vi "Prins FIFO Scheduler.vi"(8 "Number of Jobs":i32=4, 9 "Number of Machines":i32=4, 10 "Processing Times(MxJ)":u16[][](array[numeric])=[[1, 62, 270, 667], [303, 255, 170, 272], [66, 556, 373, 5], [630, 127, 187, 56]], 11 "Schedule In":u16[](array[numeric])=[6, 12, 5, 1, 10, 15, 4, 0, 14, 7, 13, 3, 2, 8, 11, 9]) -> (2 "Completion Times (MxJ)":i32[][](array[numeric]), 3 "Start Times (MxJ)":i32[][](array[numeric]))   [LabVIEW 2013, in "Scheduler.lvclass"]
uses:
  Scheduler.lvclass
  Controls/GapStructure4FIFOEngine.ctl
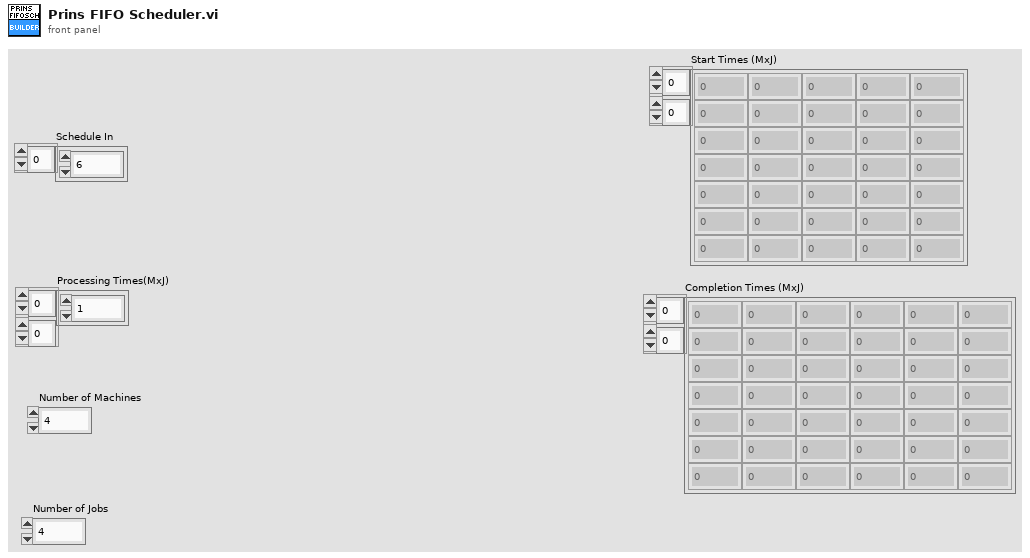
[diagram p1: front panel]
types:
  T1 = typedef "Scheduler.lvclass/GapStructure4FIFOEngine.ctl" = cluster{"Gap Start":i32, "Gap End":i32, "Gap Valid?":bool}
  T2 = typedef "Scheduler.lvclass/ValidGaps.ctl" = cluster{"Gap Start Time":i32, "Gap End Time":i32, "Gap Interval":i32}
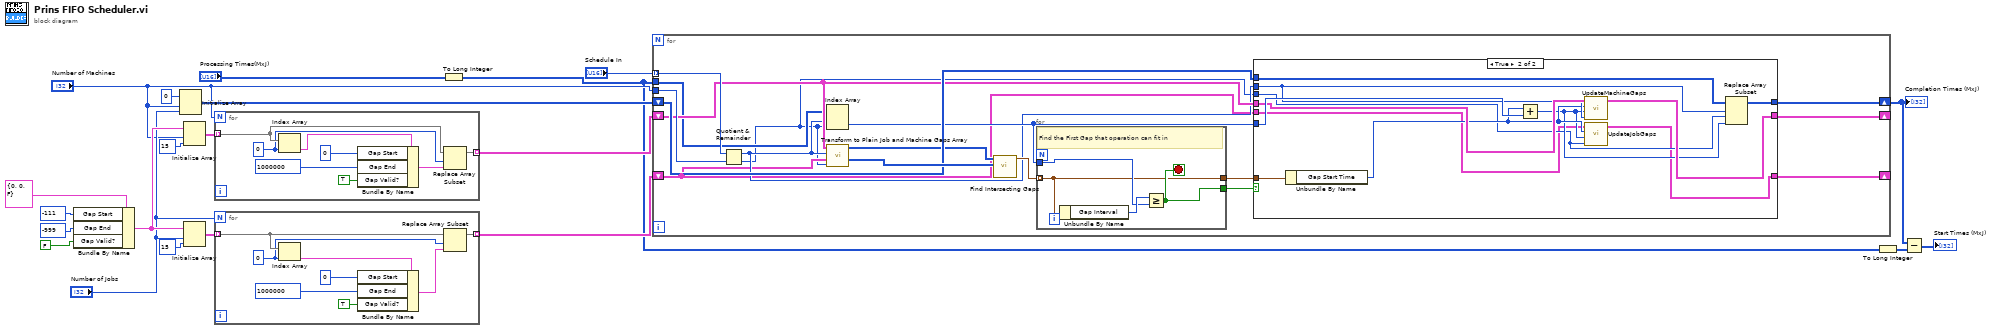
[diagram p0: block diagram]
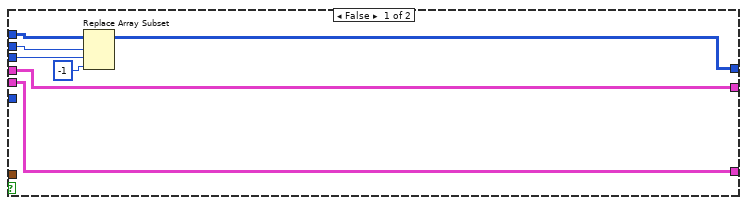
[diagram p2: hidden frame]
diagram:
  n1 = Bundle By Name(cluster=T1 {"Gap Start"=0, "Gap End"=0, "Gap Valid?"=FALSE}, "Gap Start"=-111, "Gap End"=-999, "Gap Valid?"=FALSE) -> (w13:T1)
  n2 = Initialize Array(0, "Number of Machines", "Number of Jobs") -> (w9:i32[][])
  n3 = Initialize Array(w13, "Number of Machines", 15 ("dimension size")) -> (w12:T1[][])
  n4 = Initialize Array(w13, "Number of Jobs", 15 ("dimension size")) -> (w15:T1[][])
  n5 = for {
    N: "Number of Machines" -> [_]
    tunnel: [w22] -> w11 mode=indexing
    tunnel: w12 -> [w25] mode=indexing
    w24 = 0 ("index")
    n6 = Index Array(array=w25, index=w24) -> (element=w29:T1)
    n7 = Bundle By Name(cluster=w29, "Gap Start"=0, "Gap End"=1000000, "Gap Valid?"=TRUE) -> (w23:T1)
    n8 = Replace Array Subset(array=w25, new element=w23, index=w24) -> (w22:T1[])
  }
  n9 = for {
    N: "Number of Jobs" -> [_]
    tunnel: [w30] -> w21 mode=indexing
    tunnel: w15 -> [w33] mode=indexing
    w32 = 0 ("index")
    n10 = Index Array(array=w33, index=w32) -> (element=w37:T1)
    n11 = Bundle By Name(cluster=w37, "Gap Start"=0, "Gap End"=1000000, "Gap Valid?"=TRUE) -> (w31:T1)
    n12 = Replace Array Subset(array=w33, new element=w31, index=w32) -> (w30:T1[])
  }
  n13 = To Long Integer(number="Processing Times(MxJ)") -> (32bit integer=w1:i32[][])
  n14 = for {
    tunnel: "Schedule In" -> [w54] mode=indexing
    tunnel: "Number of Machines" -> [w53]
    shift-right: [w47] -> w4
    shift-left: w9 -> [w48]
    tunnel: w1 -> [w43]
    shift-right: [w45] -> _
    shift-left: w11 -> [w46]
    shift-right: [w44] -> _
    shift-left: w21 -> [w39]
    n15 = Quotient & Remainder(x=w54, y=w53) -> (x-y*floor(x/y)=w40:i32, floor(x/y)=w38:i32)
    n16 = Index Array(array=w43, index (row)=w40, index (col)=w38) -> (element=w42:i32)
    n17 = call "Transform to Plain Job and Machine Gaps Array.vi"("v"=w38, "Job Gaps"=w39, "u"=w40, "Machine Gaps"=w46) -> ("Job Gaps Array"=w52:i32[][], "Machine Gaps Array"=w41:i32[][])  [unwired: 6 in]
    n18 = call "Find Intersecting Gaps.vi"("Job Gaps Array"=w52, "Machine Gaps Array"=w41) -> ("Gaps Array"=w51:T2[])  [unwired: 9 in]
    n19 = for {
      tunnel: w51 -> [w74] mode=indexing
      tunnel: w42 -> [w76]
      tunnel: [w75] -> w50
      tunnel: [w74] -> w49
      stop <- w75 stop-if-true
      # "Find the First Gap that operation can fit in"
      n20 = Unbundle By Name(w74) -> ("Gap Interval"=w77:i32)
      n21 = Greater Or Equal?(x=w77, y=w76) -> (x >= y?=w75:bool)
    }
    n22 = case shown="True" w50 {
      tunnel: w49 -> [_ w73]
      tunnel: w48 -> [w56 w72]
      tunnel: w40 -> [w59 w67]
      tunnel: w38 -> [w58 w64]
      tunnel: w42 -> [_ w71]
      tunnel: [w55 w70] -> w47
      tunnel: w46 -> [w61 w68]
      tunnel: [w61 w69] -> w45
      tunnel: w39 -> [w60 w63]
      tunnel: [w60 w62] -> w44
      frame False {
        n23 = Replace Array Subset(array=w56, new element=-1 ("new element/subarray"), index (row)=w59, index (col)=w58) -> (w55:i32[][])
      }
      frame True {
        n24 = Unbundle By Name(w73) -> ("Gap Start Time"=w66:i32)
        n25 = Add(x=w66, y=w71) -> (x+y=w65:i32)
        n26 = call "UpdateMachineGaps.vi"("u( Machine Index)"=w67, "Operation Finish Time"=w65, "Operation Start Time"=w66, "Machine Gaps in"=w68) -> ("Machine Gaps out"=w69:T1[][])  [unwired: 7 in]
        n27 = call "UpdateJobGaps.vi"("v( Job Index)"=w64, "Operation Finish Time"=w65, "Operation Start Time"=w66, "Job Gaps in"=w63) -> ("Job Gaps out"=w62:T1[][])  [unwired: 7 in]
        n28 = Replace Array Subset(array=w72, new element=w65, index (row)=w67, index (col)=w64) -> (w70:i32[][])
      }
    }
  }
  "Completion Times (MxJ)" <- w4
  n29 = To Long Integer(number=w1) -> (32bit integer=w3:i32[][])
  n30 = Subtract(x=w4, y=w3) -> (x-y=→"Start Times (MxJ)":i32[][])
